vi "create ref.vi"(8 "error in (no error)":errorcluster, 9 "Image Name":string="untitled", 11 "MeritFactor in":refnum<class "MeritFactor.lvclass">) -> (0 "error out":errorcluster, 3 "MeritFactor out":refnum<class "MeritFactor.lvclass">)   [LabVIEW 2012, in "MeritFactor.lvclass"]
uses:
  MeritFactor.lvclass
  MeritFactor.lvclass/MeritFactor.ctl
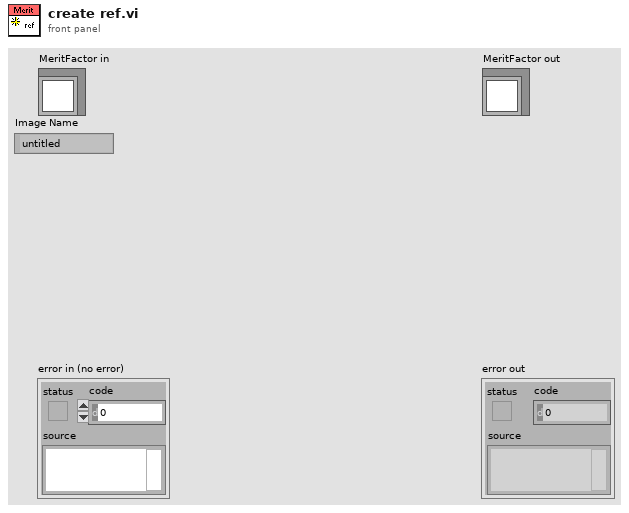
[diagram p1: front panel]
types:
  T1 = typedef "Image Type" = u32
  T2 = typedef "IMAQ Image.ctl" = refnum<image>
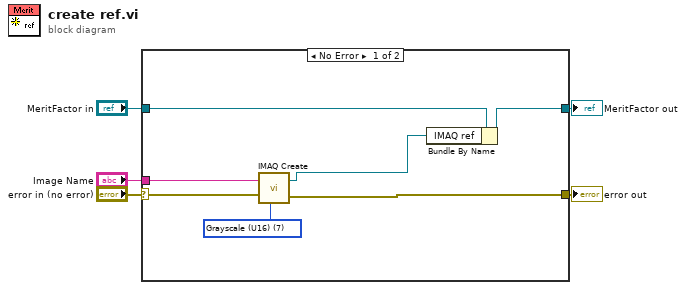
[diagram p0: block diagram]
diagram:
  n1 = case shown="No Error" "error in (no error)" {
    selector: "error in (no error)" -> [w10 w14]
    tunnel: [w7 w14] -> w4
    tunnel: "Image Name" -> [w11 _]
    tunnel: "MeritFactor in" -> [w9 w13]
    tunnel: [w8 w13] -> w1
    frame No Error {
      w12 = T1 7 items=["Grayscale (U8)", "Grayscale (I16)", "Grayscale (SGL)", "Complex (CSG)", "RGB (U32)", "HSL (U32)", "RGB (U64)", "Grayscale (U16)"] ("Image Type")
      n2 = call "IMAQ Create"("Image Name"=w11, "Image Type"=w12, "error in (no error)"=w10) -> ("New Image"=w6:T2, "error out"=w7:errorcluster)  [unwired: 2 in]
      n3 = Bundle By Name(cluster=w9, "IMAQ ref"=w6) -> (w8:refnum<class "MeritFactor.lvclass">)
    }
    frame Error {
    }
  }
  "error out" <- w4
  "MeritFactor out" <- w1
